vi "Compare.vi"(1 "z2":dbl, 2 "z1":dbl) -> (0 "Boolean":bool)   [LabVIEW 2025]
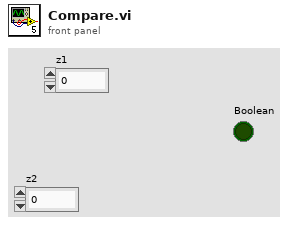
[diagram p1: front panel]
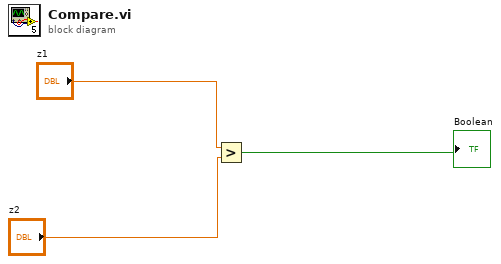
[diagram p0: block diagram]
diagram:
  n1 = Greater?(x="z1", y="z2") -> (0:→"Boolean":bool)
